vi "dvp Vi Get Black Level.vi"(10 "pBlackLevel":sgl, 11 "handle":u32) -> (2 "pBlackLevel out":sgl, 3 "function return":u32(ring))   [LabVIEW 2018, in "LabViewDVPCamera.lvlib"]
doc: "LabviewDvp2Api dvpStatus dvpViGetBlackLevel(dvpHandle handle, float *pBlackLevel);"
uses:
  LabViewDVPCamera.lvlib
  LabViewDVPCamera/LabViewDVPCamera.dll
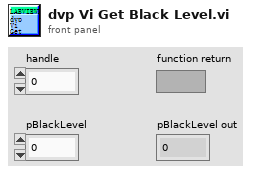
[diagram p1: front panel]
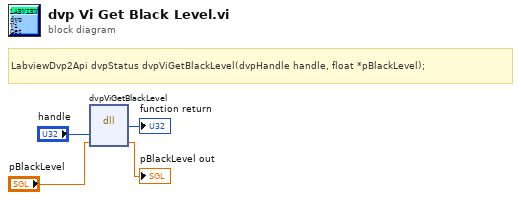
[diagram p0: block diagram]
diagram:
  # "LabviewDvp2Api dvpStatus dvpViGetBlackLevel(dvpHandle handle, float *pBlackLevel);"
  n1 = dll-call lib="C:/Program Files (x86)/DVP2 Labview cn 64/Sample/LabViewDVPCamera/LabViewDVPCamera.*" fn="dvpViGetBlackLevel"("handle"="handle", "pBlackLevel"="pBlackLevel") -> (→"function return":u32, "pBlackLevel"=→"pBlackLevel out":sgl)  [unwired: 4 in, 2 out]
